vi "RSP_EnterFATMode.vi"(0 "Error In":errorcluster, 1 "Response":u8[](array[numeric]) format="%x") -> (2 "Status":bool, 3 "Error Out":errorcluster, 4 "Generic_Mimic_Data":T1)   [LabVIEW 2014]
uses:
  MIMIC_ResponseCluster.ctl
panel:
  # "Enter FAT Mode Response:"
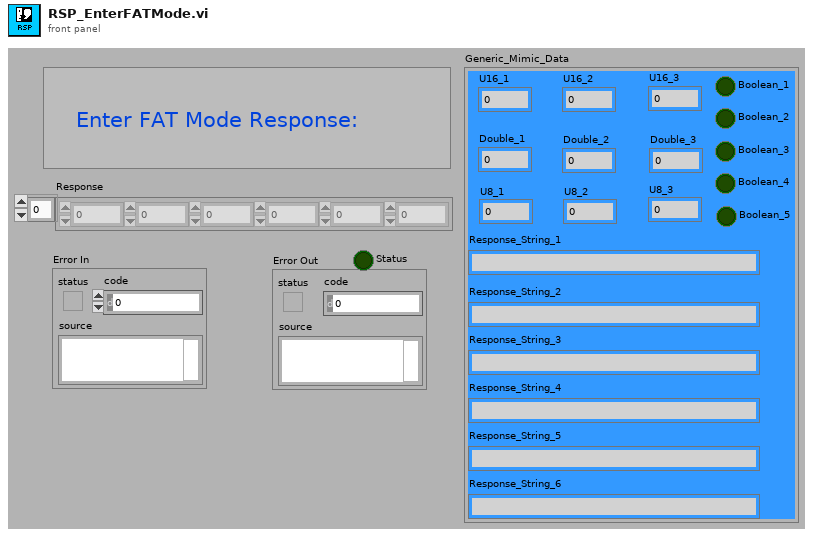
[diagram p1: front panel]
types:
  T1 = typedef "MIMIC_ResponseCluster.ctl" = cluster{"Response_String_1":string, "Response_String_2":string, "Response_String_3":string, "Response_String_4":string, "Response_String_5":string, "Response_String_6":string, "U16_1":u16, "Boolean_1":bool, "Boolean_2":bool, "Boolean_3":bool, "Boolean_4":bool, "Boolean_5":bool, "U16_2":u16, "U16_3":u16, "Double_1":dbl, "Double_2":dbl, "Double_3":dbl, "U8_1":dbl, "U8_2":dbl, "U8_3":dbl}
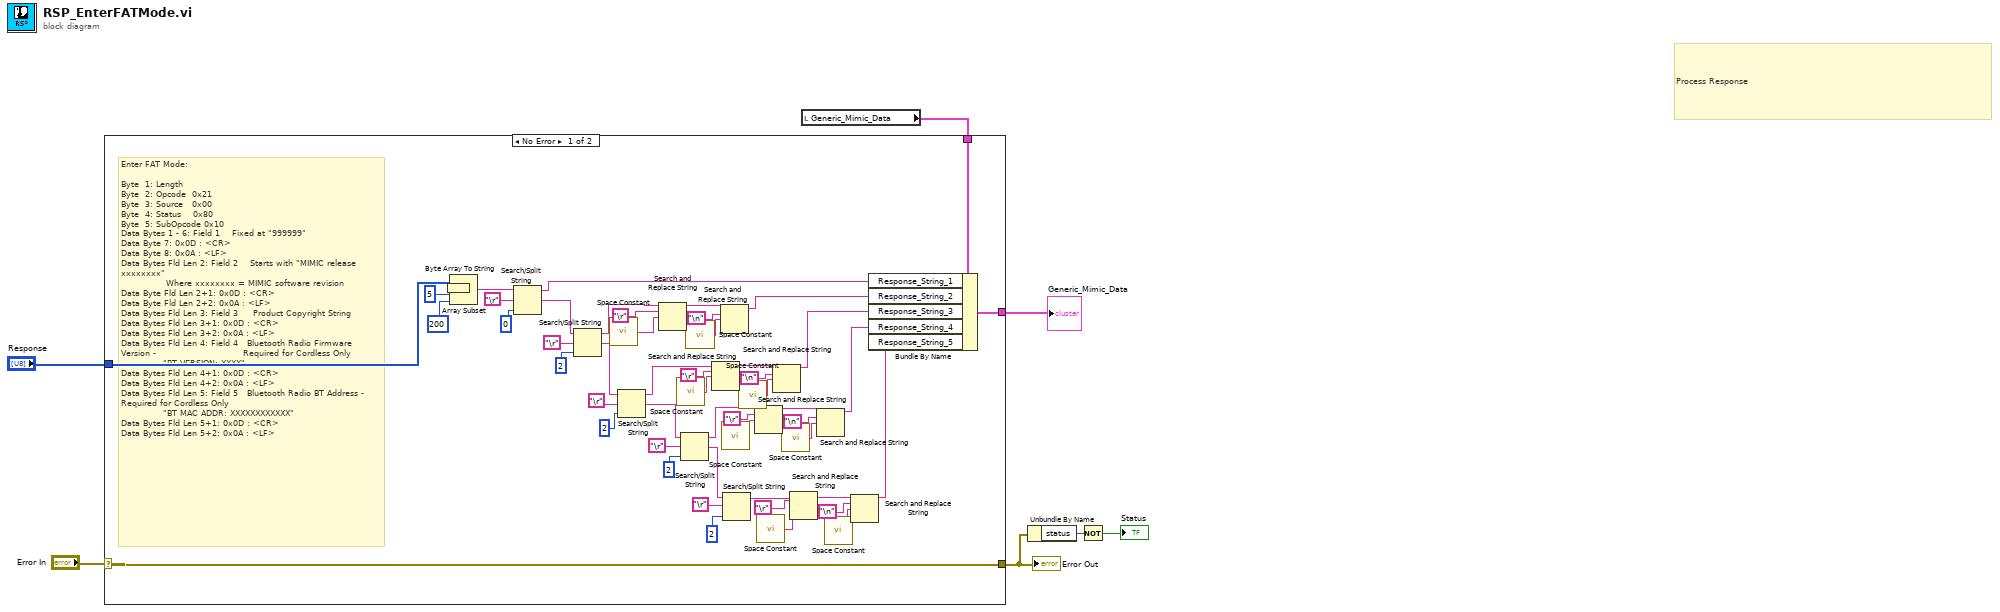
[diagram p0: block diagram]
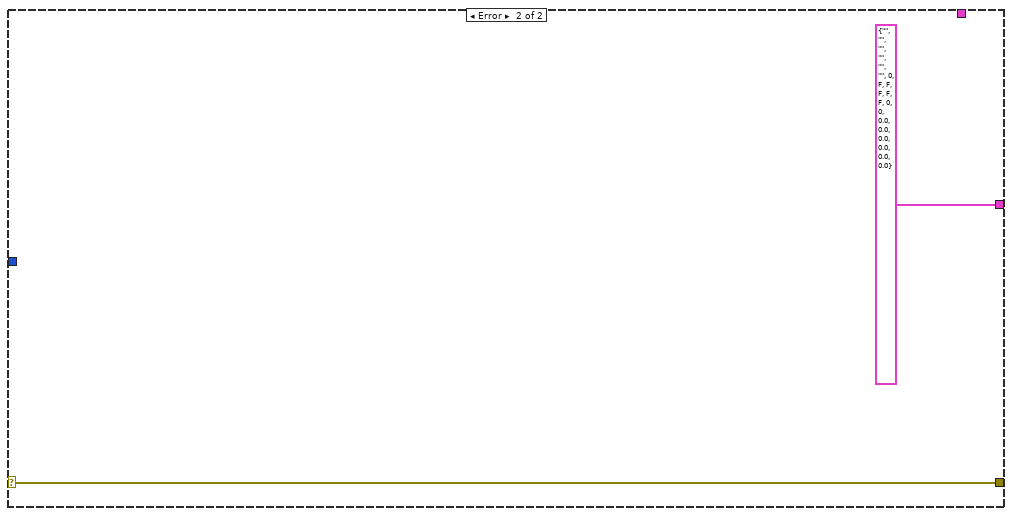
[diagram p2: hidden frame]
diagram:
  # "Process Response"
  n1 = local read "Generic_Mimic_Data"() -> (w2:T1)
  n2 = case shown="No Error" "Error In" {
    selector: "Error In" -> [w58 w60]
    tunnel: [w58 w60] -> w6
    tunnel: "Response" -> [w10 _]
    tunnel: w2 -> [w9 _]
    tunnel: [w8 T1 {"Response_String_1"="", "Response_String_2"="", "Response_String_3"="", "Response_String_4"="", "Response_String_5"="", "Response_String_6"="", "U16_1"=0, "Boolean_1"=FALSE, "Boolean_2"=FALSE, "Boolean_3"=FALSE, "Boolean_4"=FALSE, "Boolean_5"=FALSE, "U16_2"=0, "U16_3"=0, "Double_1"=0.0, "Double_2"=0.0, "Double_3"=0.0, "U8_1"=0.0, "U8_2"=0.0, "U8_3"=0.0} ("Generic_Mimic_Data")] -> w1
    frame No Error {
      # "Enter FAT Mode:\n\nByte  1: Length\nByte  2: Opcode  0x21 \nByte  3: Source   0x00\nByte  4: Status    0x80\nByte  5: SubOpcode 0x10\nData Bytes 1 - 6:\tField 1    Fixed at \"999999\"\nData Byte 7:\t0x0D : <CR>\nData Byte 8:\t0x0A : <LF>\nData Bytes Fld Len 2:\tField 2    Starts with \"MIMIC release xxxxxxxx\"\n               Where xxxxxxxx = MIMIC software revision\nData Byte Fld Len 2+1:\t0x0D : <CR>\nData Byte Fld Len 2+2:\t0x0A : <LF>\nData Bytes Fld Len 3:\tField 3     Product Copyright String\nData Bytes Fld Len 3+1:\t0x0D : <CR>\nData Bytes Fld Len 3+2:\t0x0A : <LF>\nData Bytes Fld Len 4:\tField 4   Bluetooth Radio Firmware Version -                             Required for Cordless Only          \n              \"BT VERSION: XXXX\" \nData Bytes Fld Len 4+1:\t0x0D : <CR>\nData Bytes Fld Len 4+2:\t0x0A : <LF>\nData Bytes Fld Len 5:\tField 5   Bluetooth Radio BT Address -                                       Required for Cordless Only          \n              \"BT MAC ADDR: XXXXXXXXXXXX\" \nData Bytes Fld Len 5+1:\t0x0D : <CR>\nData Bytes Fld Len 5+2:\t0x0A : <LF>"
      n3 = Array Subset(array=w10, index=5, length=200) -> (w57:u8[])
      n4 = Byte Array To String(unsigned byte array=w57) -> (string=w43:string)
      n5 = Search/Split String(string=w43, search string/char (-)="\r", offset (0)=0) -> (substring before match=w44:string, match + rest of string=w45:string)  [unwired: 1 out]
      n6 = Search/Split String(string=w45, search string/char (-)="\r", offset (0)=2) -> (substring before match=w46:string, match + rest of string=w47:string)  [unwired: 1 out]
      n7 = call <vilib>:"Space Constant.vi"() -> ("String"=w36:string)
      n8 = Search/Split String(string=w47, search string/char (-)="\r", offset (0)=2) -> (substring before match=w48:string, match + rest of string=w49:string)  [unwired: 1 out]
      n9 = Search and Replace String(input string=w46, search string="\r", replace string=w36) -> (result string=w38:string)  [unwired: 5 in, 3 out]
      n10 = call <vilib>:"Space Constant.vi"() -> ("String"=w28:string)
      n11 = Search/Split String(string=w49, search string/char (-)="\r", offset (0)=2) -> (substring before match=w50:string, match + rest of string=w51:string)  [unwired: 1 out]
      n12 = call <vilib>:"Space Constant.vi"() -> ("String"=w33:string)
      n13 = Search and Replace String(input string=w48, search string="\r", replace string=w28) -> (result string=w30:string)  [unwired: 5 in, 3 out]
      n14 = Search and Replace String(input string=w38, search string="\n", replace string=w33) -> (result string=w35:string)  [unwired: 5 in, 3 out]
      n15 = call <vilib>:"Space Constant.vi"() -> ("String"=w20:string)
      n16 = Search/Split String(string=w51, search string/char (-)="\r", offset (0)=2) -> (substring before match=w52:string)  [unwired: 2 out]
      n17 = call <vilib>:"Space Constant.vi"() -> ("String"=w25:string)
      n18 = Search and Replace String(input string=w50, search string="\r", replace string=w20) -> (result string=w22:string)  [unwired: 5 in, 3 out]
      n19 = call <vilib>:"Space Constant.vi"() -> ("String"=w13:string)
      n20 = Search and Replace String(input string=w30, search string="\n", replace string=w25) -> (result string=w27:string)  [unwired: 5 in, 3 out]
      n21 = call <vilib>:"Space Constant.vi"() -> ("String"=w17:string)
      n22 = Search and Replace String(input string=w52, search string="\r", replace string=w13) -> (result string=w53:string)  [unwired: 5 in, 3 out]
      n23 = Search and Replace String(input string=w22, search string="\n", replace string=w17) -> (result string=w19:string)  [unwired: 5 in, 3 out]
      n24 = call <vilib>:"Space Constant.vi"() -> ("String"=w12:string)
      n25 = Search and Replace String(input string=w53, search string="\n", replace string=w12) -> (result string=w54:string)  [unwired: 5 in, 3 out]
      n26 = Bundle By Name(cluster=w9, "Response_String_1"=w44, "Response_String_2"=w35, "Response_String_3"=w27, "Response_String_4"=w19, "Response_String_5"=w54) -> (w8:T1)
    }
    frame Error {
    }
  }
  "Error Out" <- w6
  "Generic_Mimic_Data" <- w1
  n27 = Unbundle By Name(w6) -> ("status"=w5:bool)
  n28 = Not(x=w5) -> (.not. x?=→"Status":bool)
